vi "DriveExecuteTestFeedFoward.vi"(8 "error in (no error)":errorcluster) -> (0 "error out":errorcluster)   [LabVIEW 2023]
doc: "Execute and test/tune feed foward for Drive\n\nClosed control loop for drive\n\ninput: \n error in (cluster)\n\noutput:\n error out (cluster)"
uses:
  <vilib>/Rock Robotics/WPI/ThirdParty/Phoenix-LabVIEW/Motor Controller/Controls/CTRE_Phoenix_MotorControl_ControlMode.ctl
  DriveGlobal.vi
  <vilib>/Rock Robotics/WPI/ThirdParty/JAS_Junk/TrajLib/Trajectory_Library.lvlib
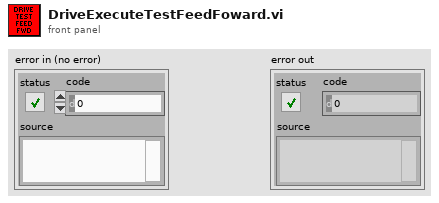
[diagram p1: front panel]
types:
  T1 = typedef "CTRE_Phoenix_MotorControl_ControlMode.ctl" = u16
  T2 = typedef "ADIS16470 Device Reference.ctl" = cluster{"DevStatus":errorcluster, "Hardware Config":T3, "Calibration Complete":refnum<notifier>, "Status Reference":refnum<data-value>, "Data Reference":refnum<data-value>, "Sychronous Process VI":T7, "Cmd FIFO":refnum<k33>, "Source":T8, "Data FIFO":refnum<k33>, "Calibration Time (ms)":u32, "Data Reference":refnum<data-value>}
  T3 = typedef "ADIS16470 Hardware Configuration.ctl" = cluster{"SPI Clock Rate (Hz)":dbl, "IMU SPI Mode (3)":T4, "IMU Reset Pin":T5, "IMU SPI Bus":T6, "IMU Data Ready Pin":T5, "Stall Config":cluster{"Pow2BytesPerRead":u8, "StallTicks":u16, "CsToSclkTicks":u8}}
  T4 = typedef "WPI_SPIMode.ctl" = enum16{"Mode 0 (Clk Idle Low,Sample on Leading)", "Mode 1 (Clk Idle Low,Sample on Trailing)", "Mode 2 (Clk Idle High,Sample on Leading)", "Mode 3 (Clk Idle High,Sample on Trailing)"}
  T5 = typedef "FPGA_DIOChannel.ctl" = enum8{"DIO 0", "DIO 1", "DIO 2", "DIO 3", "DIO 4", "DIO 5", "DIO 6", "DIO 7", "DIO 8", "DIO 9", "DIO MXP 0", "DIO MXP 1", "DIO MXP 2", "DIO MXP 3", "DIO MXP 4", "DIO MXP 5", "DIO MXP 6", "DIO MXP 7", "DIO MXP 8", "DIO MXP 9", "DIO MXP 10", "DIO MXP 11", "DIO MXP 12", "DIO MXP 13", "DIO MXP 14", "DIO MXP 15", "SPI Port CS1", "SPI Port CS2", "SPI Port CS3", "SPI Port MISO", "SPI Port MOSI", "Invalid"}
  T6 = typedef "spi_bus.ctl" = enum16{"SPI On-Board, CS0", "SPI On-Board, CS1", "SPI On-Board, CS2", "SPI On-Board, CS3", "SPI MXP", "Invalid"}
  T7 = typedef "ADIS16470 Process.ctl" = refnum<vi>
  T8 = typedef "FPGA_CounterEncoderSourceConvertionLVSourceType.ctl" = cluster{"DevStatus":errorcluster, "AnalogTriggerMode?":bool, "DigitalMode":cluster{"DIO Channel":T9}, "AnalogTriggerMode":cluster{"AnalogTriggerIndex":T10, "OutputType":T11}}
  T9 = typedef "FPGA_DIODigitalSourceChannel.ctl" = enum8{"DIO 0", "DIO 1", "DIO 2", "DIO 3", "DIO 4", "DIO 5", "DIO 6", "DIO 7", "DIO 8", "DIO 9", "DIO MXP 0", "DIO MXP 1", "DIO MXP 2", "DIO MXP 3", "DIO MXP 4", "DIO MXP 5", "DIO MXP 6", "DIO MXP 7", "DIO MXP 8", "DIO MXP 9", "DIO MXP 10", "DIO MXP 11", "DIO MXP 12", "DIO MXP 13", "DIO MXP 14", "DIO MXP 15", "SPI Port CS1", "SPI Port CS2", "SPI Port CS3", "SPI Port MISO", "SPI Port MOSI", "Disabled"}
  T10 = typedef "FPGA_AnalogTriggerIndex.ctl" = enum8{"Trig 0", "Trig 1", "Trig 2", "Trig 3", "Trig 4", "Trig 5", "Trig 6", "Trig 7", "Invalid"}
  T11 = typedef "FPGA_AnalogTriggerOutType.ctl" = enum16{"InWindow", "TriggerState", "Rising", "Falling"}
  T12 = typedef "ADIS16470 Data.ctl" = cluster{"XAngle":dbl, "YAngle":dbl, "ZAngle":dbl}
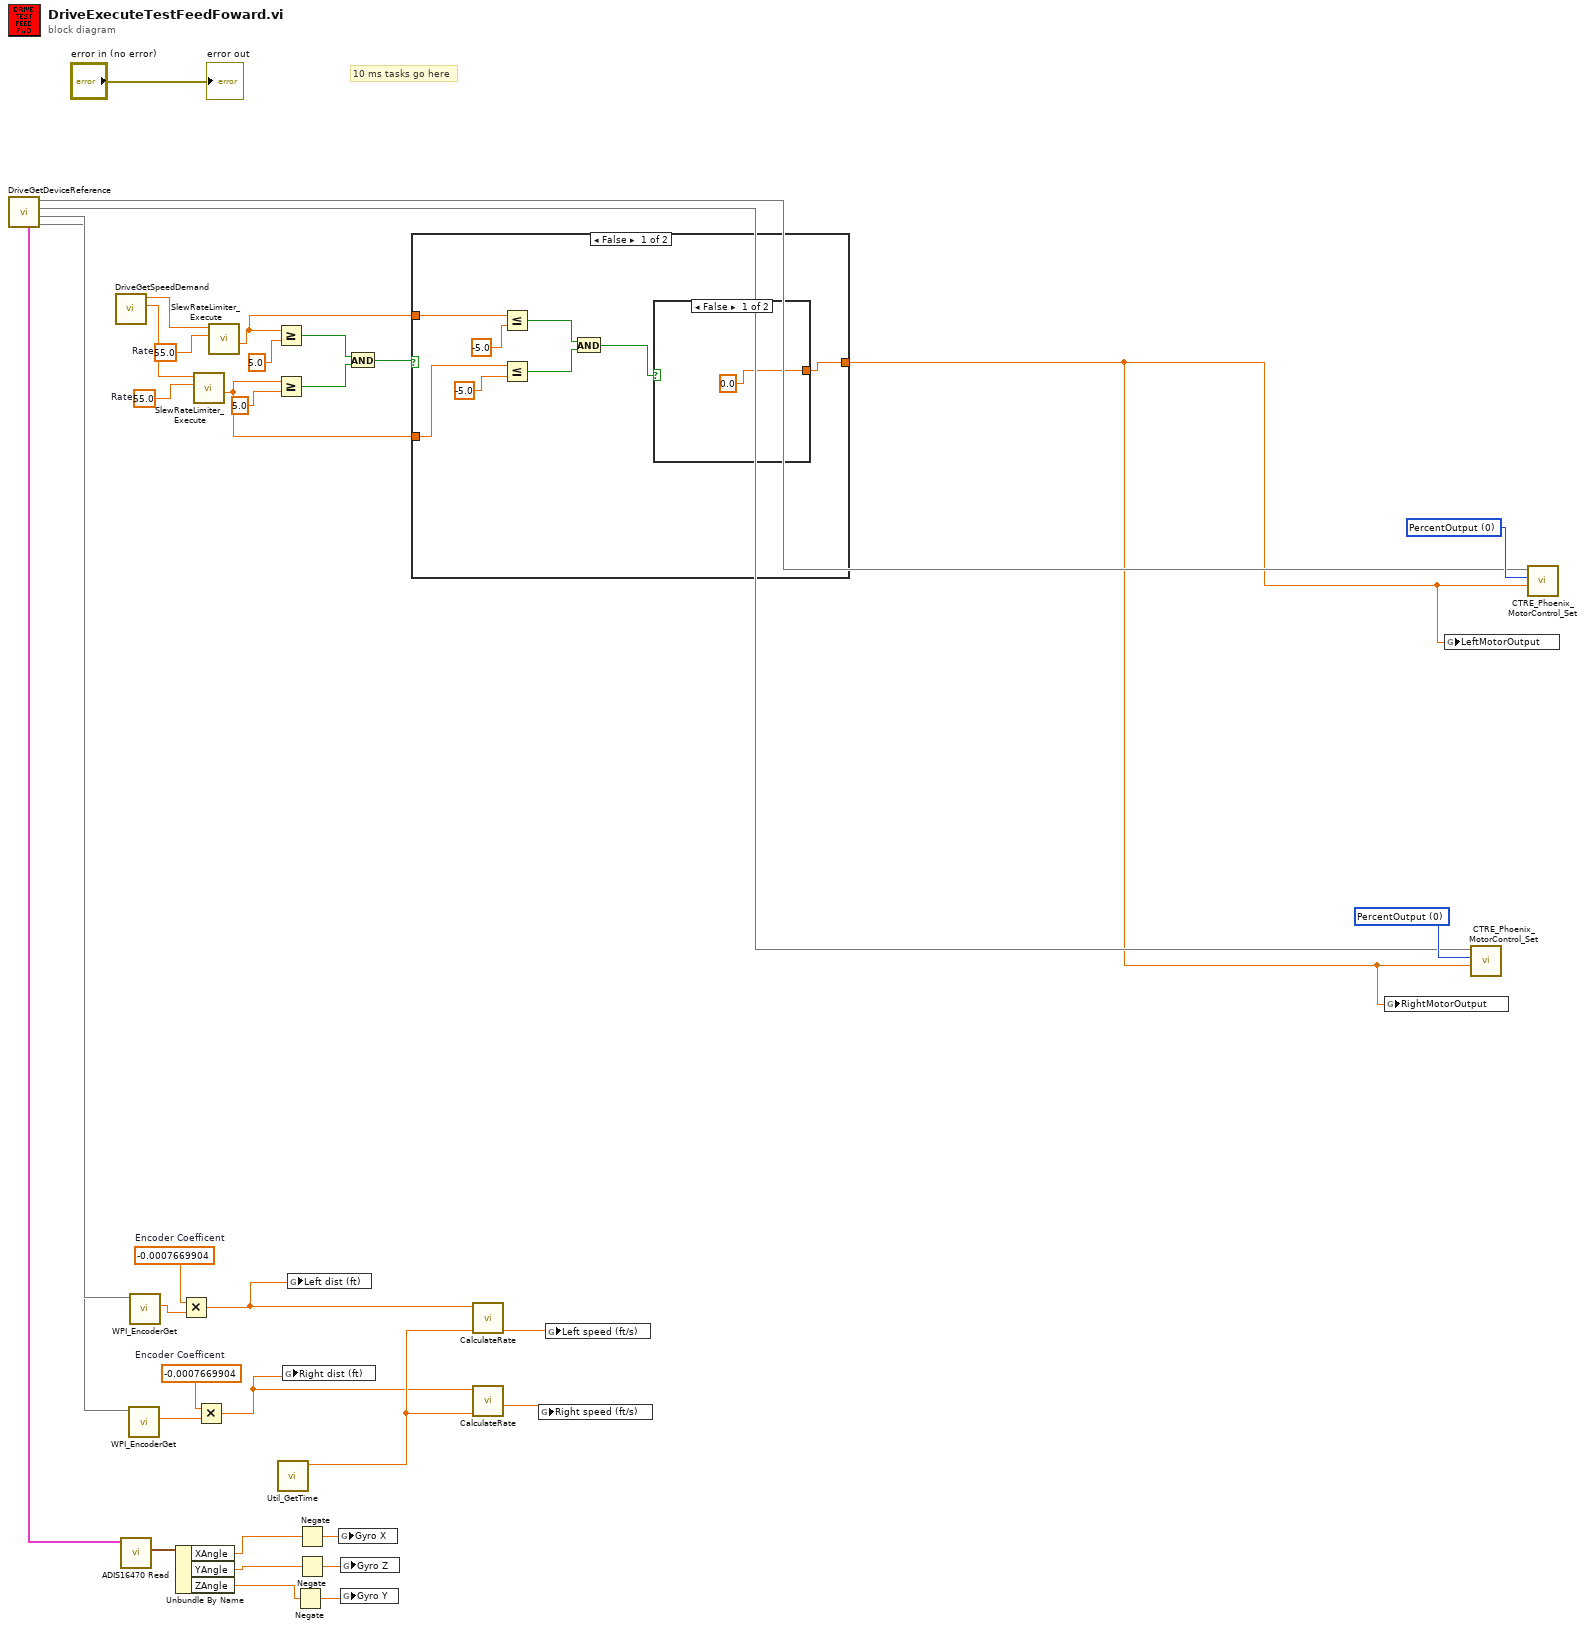
[diagram p0: block diagram]
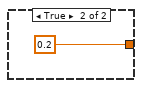
[diagram p2: hidden frame]
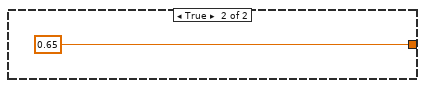
[diagram p3: hidden frame]
diagram:
  w7 = -0.0007669904  # Encoder Coefficent
  w8 = -0.0007669904  # Encoder Coefficent
  w24 = 55.0  # Rate
  w26 = 55.0  # Rate
  w35 = T1 0 items=["PercentOutput"=0, "Position"=1, "Velocity"=2, "Current"=3, "Follower"=5, "MotionProfile"=6, "MotionMagic"=7, "MotionProfileArc"=10, "Disabled"=15] ("Control Mode")
  w36 = T1 0 items=["PercentOutput"=0, "Position"=1, "Velocity"=2, "Current"=3, "Follower"=5, "MotionProfile"=6, "MotionMagic"=7, "MotionProfileArc"=10, "Disabled"=15] ("Control Mode")
  # "10 ms tasks go here"
  n1 = call "DriveGetDeviceReference.vi"() -> (0:w3, 1:w4, 2:w27, 3:w28, "Gryo"=w32:T2)  [unwired: 7 in]
  n2 = call "DriveGetSpeedDemand.vi"() -> ("vY"=w23:dbl, "vX"=w25:dbl)  [unwired: 8 in, 2 out]
  n3 = call <vilib>:"ADIS16470 Read.vi"("ADIS16470DevRef"=w32) -> ("ADIS16470 Value"=w33:T12)  [unwired: 7 in, 3 out]
  n4 = call <vilib>:"WPI_EncoderGet.vi"("EncoderDevRef"=w3) -> ("Distance"=w5:dbl)  [unwired: 5 in, 5 out]
  n5 = call <vilib>:"WPI_EncoderGet.vi"("EncoderDevRef"=w4) -> ("Distance"=w6:dbl)  [unwired: 5 in, 5 out]
  n6 = Unbundle By Name(w33) -> ("XAngle"=w17:dbl, "YAngle"=w19:dbl, "ZAngle"=w18:dbl)
  n7 = Multiply(x=w8, y=w6) -> (x*y=w1:dbl)
  n8 = call <vilib>:"SlewRateLimiter_Execute.vi"("PositiveRate"=w24, "Input"=w23) -> ("Output"=w9:dbl)  [unwired: 8 in, 1 out]
  n9 = Multiply(x=w7, y=w5) -> (x*y=w2:dbl)
  n10 = call <vilib>:"SlewRateLimiter_Execute.vi"("PositiveRate"=w26, "Input"=w25) -> ("Output"=w10:dbl)  [unwired: 8 in, 1 out]
  n11 = Greater Or Equal?(x=w10, y=5.0) -> (x >= y?=w14:bool)
  n12 = Greater Or Equal?(x=w9, y=5.0) -> (x >= y?=w13:bool)
  n13 = call <vilib>:"Util_GetTime.vi"() -> ("FPGA_Time_Seconds"=w31:dbl)  [unwired: 9 in, 2 out]
  n14 = global write "DriveGlobal.vi" "Right dist (ft)"(w2) -> ()
  n15 = global write "DriveGlobal.vi" "Left dist (ft)"(w1) -> ()
  n16 = Negate(x=w18) -> (-x=w21:dbl)
  n17 = Negate(x=w17) -> (-x=w22:dbl)
  n18 = Negate(x=w19) -> (-x=w20:dbl)
  n19 = global write "DriveGlobal.vi" "Gyro X"(w22) -> ()
  n20 = global write "DriveGlobal.vi" "Gyro Z"(w20) -> ()
  n21 = global write "DriveGlobal.vi" "Gyro Y"(w21) -> ()
  n22 = And(x=w14, y=w13) -> (x .and. y?=w12:bool)
  n23 = case shown="False" w12 {
    tunnel: [w37 0.65] -> w11
    tunnel: w10 -> [w40 _]
    tunnel: w9 -> [w39 _]
    frame False {
      n24 = Less Or Equal?(x=w40, y=-5.0) -> (x <= y?=w43:bool)
      n25 = Less Or Equal?(x=w39, y=-5.0) -> (x <= y?=w44:bool)
      n26 = And(x=w43, y=w44) -> (x .and. y?=w38:bool)
      n27 = case shown="False" w38 {
        tunnel: [0.0 0.2] -> w37
        frame False {
        }
        frame True {
        }
      }
    }
    frame True {
    }
  }
  n28 = call "CalculateRate.vi"("Time (s)"=w31, "Distance (units)"=w1) -> ("Rate (units/s)"=w30:dbl)  [unwired: 9 in]
  n29 = call "CalculateRate.vi"("Time (s)"=w31, "Distance (units)"=w2) -> ("Rate (units/s)"=w29:dbl)  [unwired: 9 in]
  n30 = global write "DriveGlobal.vi" "Right speed (ft/s)"(w29) -> ()
  n31 = global write "DriveGlobal.vi" "Left speed (ft/s)"(w30) -> ()
  n32 = global write "DriveGlobal.vi" "RightMotorOutput"(w11) -> ()
  n33 = global write "DriveGlobal.vi" "LeftMotorOutput"(w11) -> ()
  n34 = call <vilib>:"CTRE_Phoenix_MotorControl_Set.vi"("Output"=w11, "Control Mode"=w35, "PhoenixMotorControlDevRef"=w27) -> ()  [unwired: 7 in, 2 out]
  n35 = call <vilib>:"CTRE_Phoenix_MotorControl_Set.vi"("Output"=w11, "Control Mode"=w36, "PhoenixMotorControlDevRef"=w28) -> ()  [unwired: 7 in, 2 out]
  "error out" <- "error in (no error)"
